vi "Update Assert Data.vi"(8 "error in (no error)":errorcluster, 10 "Assert Packet":T1, 11 "AssertEngine in":refnum<class "AssertEngine.lvclass">) -> (0 "error out":errorcluster, 3 "AssertEngine out":refnum<class "AssertEngine.lvclass">)   [LabVIEW 2016, in "AssertEngine.lvlib" / "AssertEngine.lvclass"]
doc: "Updates the arrays of assert names (Assert List) and the parameters for each (Values)."
uses:
  AssertEngine.lvclass
  Assert Packet.ctl
  Log Assert/Assert Data.ctl
  AssertEngine.lvclass/AssertEngine.ctl
  AssertEngine.lvlib
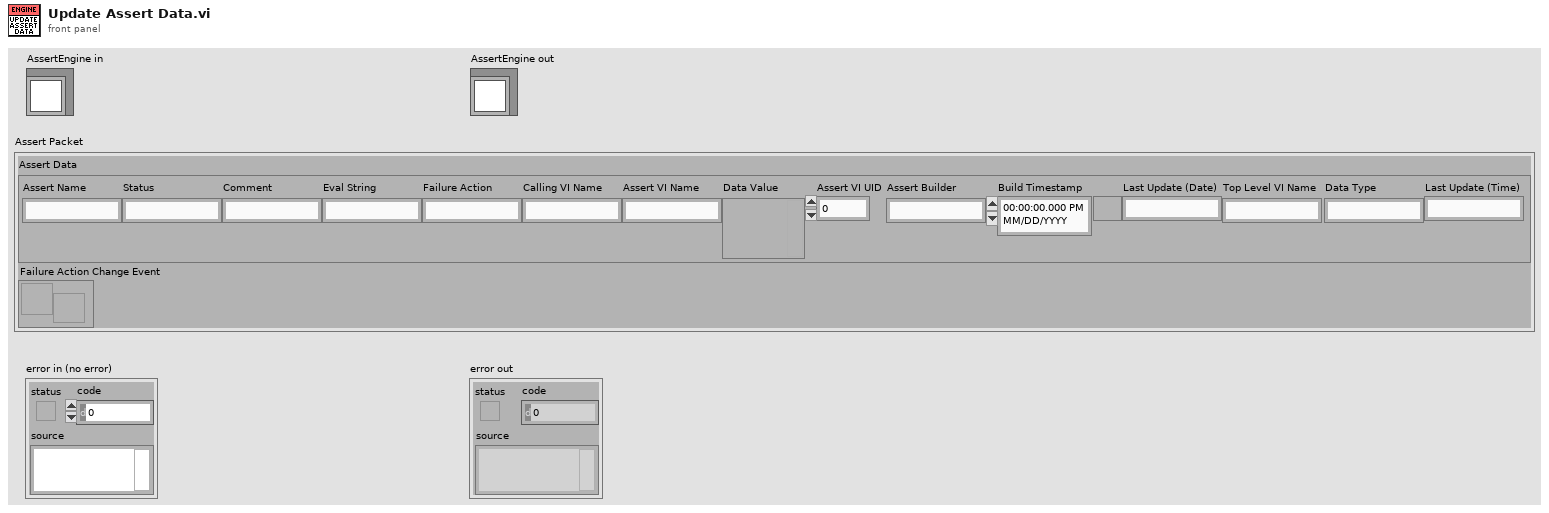
[diagram p1: front panel]
types:
  T1 = typedef "AssertEngine.lvlib/AssertEngine.lvclass/Assert Packet.ctl" = cluster{"Assert Data":T2, "Failure Action Change Event":refnum<user-event>}
  T2 = typedef "AssertEngine.lvlib/Assert Data.ctl" = cluster{"Assert Name":string, "Status":string, "Comment":string, "Eval String":string, "Failure Action":string, "Calling VI Name":string, "Assert VI Name":string, "Data Value":variant, "Assert VI UID":i32, "Assert Builder":string, "Build Timestamp":timestamp, "Last Update (Date)":string, "Top Level VI Name":string, "Data Type":string, "Last Update (Time)":string}
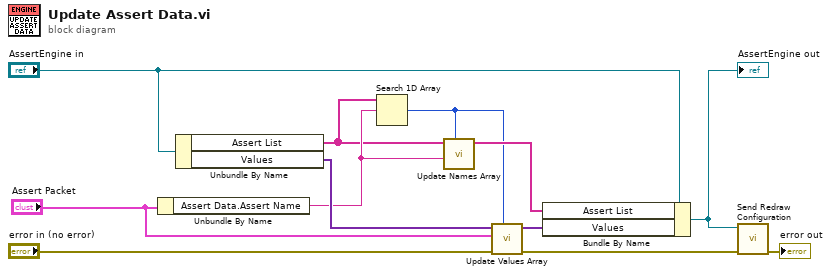
[diagram p0: block diagram]
diagram:
  n1 = Unbundle By Name("Assert Packet") -> ("Assert Data.Assert Name"=w5:string)
  n2 = Unbundle By Name("AssertEngine in") -> ("Assert List"=w3:string[], "Values"=w11:variant[])
  n3 = Search 1D Array(1D array=w3, element=w5) -> (index of element=w2:i32)  [unwired: 1 in]
  n4 = call "Update Names Array.vi"("index of element"=w2, "Assert Data"=w5, "Assert List in"=w3) -> ("Assert List out"=w4:string[])  [unwired: 8 in]
  n5 = call "Update Values Array.vi"("index of element"=w2, "error in (no error)"="error in (no error)", "Assert Packet"="Assert Packet", "Values in"=w11) -> ("error out"=w9:errorcluster, "Values out"=w8:variant[])  [unwired: 6 in]
  n6 = Bundle By Name(cluster="AssertEngine in", "Assert List"=w4, "Values"=w8) -> (w6:refnum<class "AssertEngine.lvclass">)
  "AssertEngine out" <- w6
  n7 = call "Send Redraw Configuration.vi"("error in (no error)"=w9, "AssertEngine in"=w6) -> ("error out"=→"error out":errorcluster)  [unwired: 9 in]
